vi "Set Event Reg.vi"(8 "error in (no error)":errorcluster, 10 "Event Reg":refnum<event-registration>, 11 "ArrayManager in":refnum<class "ArrayManager.lvclass">) -> (0 "error out":errorcluster, 3 "ArrayManager out":refnum<class "ArrayManager.lvclass">)   [LabVIEW 2014, in "OOPanel.lvlib" / "ArrayManager.lvclass"]
uses:
  ArrayManager.lvclass
  Events.ctl
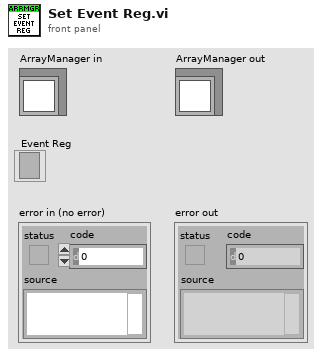
[diagram p1: front panel]
types:
  T1 = typedef "OOPanel.lvlib/ArrayManager.lvclass/Event Regs.ctl" = cluster{"Event Reg":refnum<event-registration>, "Last Update Ticks ms":u32}
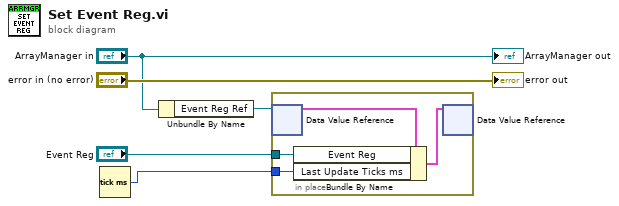
[diagram p0: block diagram]
diagram:
  n1 = Tick Count (ms)() -> (millisecond timer value=w1:u32)
  n2 = Unbundle By Name("ArrayManager in") -> ("Event Reg Ref"=w4:refnum<data-value>)
  n3 = in-place {
    in-place-border: "Event Reg" -> [w7]
    in-place-border: w1 -> [w6]
    n4 = in-place-dvr #1(w4) -> (w9:T1)  [unwired: 1 out]
    n5 = Bundle By Name(cluster=w9, "Event Reg"=w7, "Last Update Ticks ms"=w6) -> (w8:T1)
    n6 = in-place-dvr #1(w8) -> ()  [unwired: 2 out]
  }
  "error out" <- "error in (no error)"
  "ArrayManager out" <- "ArrayManager in"
